vi "Run.vi"(7 "Team Index":i32, 8 "Column":i32, 9 "Row":i32, 10 "View":i32[](array[numeric]) caption="View (Team Index, -1: empty)", 11 "64 In":refnum<class "Picture.lvclass">) -> (0 "Replicated":refnum<class "Square.lvclass">, 1 "Direction":T1, 2 "Action":T2, 3 "64 Out":refnum<class "Picture.lvclass">)   [LabVIEW 2015, in "Picture.lvclass"]
uses:
  Picture.lvclass
  Type Defs/Action Enum.ctl
  Type Defs/Direction Enum.ctl
  Square/Square.lvclass
  Picture.lvclass/Picture.ctl
  SubVIs/Read-Only Globals.vi
  SubVIs/Globals (private).vi
  Type Defs/SB Type Defs.lvlib
  Common/Common.lvlib
panel:
  # "NW\nN\nNE\nE\nSE\nS\nSW\nW"
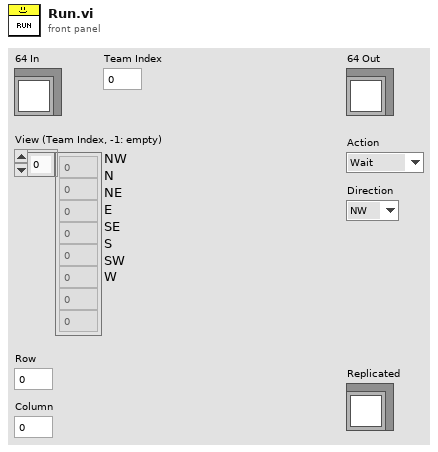
[diagram p1: front panel]
types:
  T1 = typedef "SB Type Defs.lvlib/Direction Enum.ctl" = enum16{"NW", "N", "NE", "E", "SE", "S", "SW", "W"}
  T2 = typedef "SB Type Defs.lvlib/Action Enum.ctl" = enum16{"Wait", "Move", "Attack", "Replicate"}
  T3 = typedef "Common.lvlib/Position.ctl" = cluster{"Column":i32, "Row":i32}
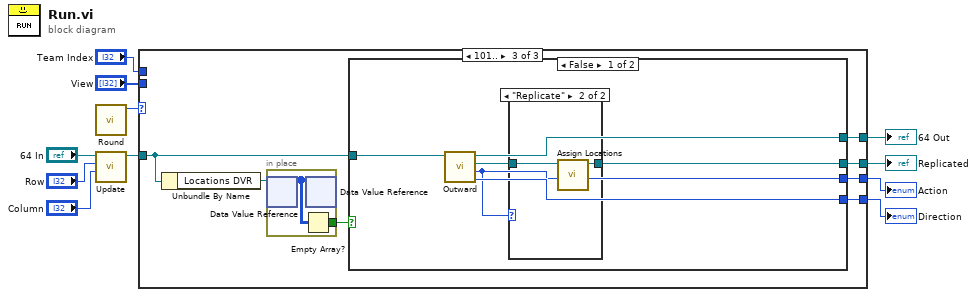
[diagram p0: block diagram]
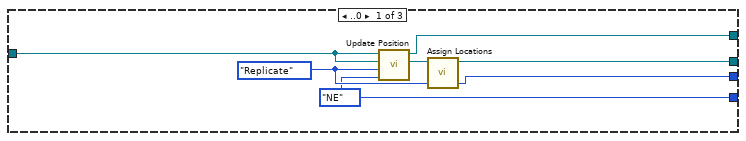
[diagram p2: hidden frame]
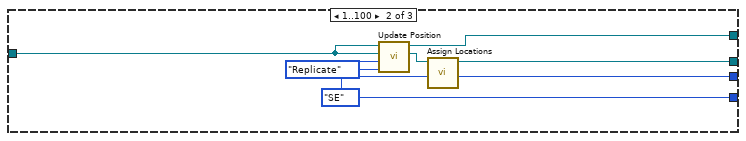
[diagram p3: hidden frame]
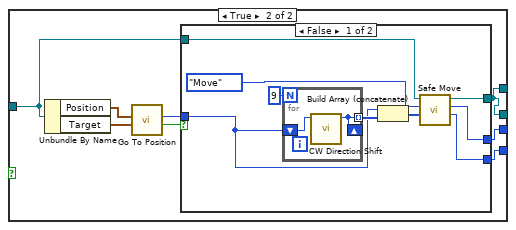
[diagram p5: hidden frame]
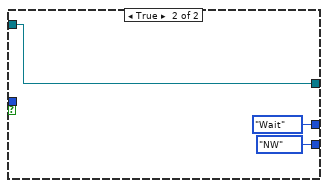
[diagram p6: hidden frame]
diagram:
  n1 = call "Round.vi"() -> ("Round"=w3:i32)  [unwired: 11 in]
  n2 = call "Update.vi"("Column"="Column", "Row"="Row", "64 in"="64 In") -> ("64 out"=w10:refnum<class "Picture.lvclass">)  [unwired: 8 in]
  n3 = case shown="101.." w3 {
    tunnel: w10 -> [w16 w22 w25]
    tunnel: [w15 w21 w30] -> w6
    tunnel: [w12 w18 w28] -> w7
    tunnel: [w14 w20 w27] -> w5
    tunnel: [w13 w19 w29] -> w4
    tunnel: "View" -> [_ _ _]
    tunnel: "Team Index" -> [_ _ _]
    frame ..0 {
      w13 = Direction_Enum."NE" ("Direction")
      w14 = Action_Enum."Replicate" ("Action")
      n4 = call "Update Position.vi"("Direction"=w13, "Action"=w14, "Replicated in"=w16, "64 in"=w16) -> ("Replicated out"=w17:refnum<class "Picture.lvclass">, "64 out"=w15:refnum<class "Picture.lvclass">)  [unwired: 6 in]
      n5 = call "Assign Locations.vi"("Picture In"=w17) -> ("Picture Out"=w12:refnum<class "Picture.lvclass">)  [unwired: 9 in, 1 out]
    }
    frame 1..100 {
      w19 = Direction_Enum."SE" ("Direction")
      w20 = Action_Enum."Replicate" ("Action")
      n6 = call "Update Position.vi"("Direction"=w19, "Action"=w20, "Replicated in"=w22, "64 in"=w22) -> ("Replicated out"=w23:refnum<class "Picture.lvclass">, "64 out"=w21:refnum<class "Picture.lvclass">)  [unwired: 6 in]
      n7 = call "Assign Locations.vi"("Picture In"=w23) -> ("Picture Out"=w18:refnum<class "Picture.lvclass">)  [unwired: 9 in, 1 out]
    }
    frame 101.. {
      n8 = Unbundle By Name(w25) -> ("Locations DVR"=w26:refnum<data-value>)
      n9 = in-place {
        in-place-border: [w62] -> w24
        n10 = in-place-dvr #1(w26) -> (w63:i32[][])  [unwired: 1 out]
        n11 = Empty Array?(array=w63) -> (empty?=w62:bool)
        n12 = in-place-dvr #1(w63) -> ()  [unwired: 2 out]
      }
      n13 = case shown="False" w24 {
        tunnel: [w36 w42] -> w30
        tunnel: [w34 w40] -> w29
        tunnel: [w33 w42] -> w28
        tunnel: [w32 w41] -> w27
        tunnel: w25 -> [w31 w43]
        frame False {
          n14 = call "Outward.vi"("64 in"=w31) -> ("Direction"=w34:i32, "Action"=w32:T2, "Replicated out"=w35:refnum<class "Picture.lvclass">, "64 out"=w36:refnum<class "Picture.lvclass">)  [unwired: 7 in]
          n15 = case shown="\"Replicate\"" w32 {
            tunnel: w35 -> [w37 w39]
            tunnel: [w37 w38] -> w33
            frame Default {
            }
            frame "Replicate" {
              n16 = call "Assign Locations.vi"("Picture In"=w39) -> ("Picture Out"=w38:refnum<class "Picture.lvclass">)  [unwired: 9 in, 1 out]
            }
          }
        }
        frame True {
          n17 = Unbundle By Name(w43) -> ("Position"=w45:T3, "Target"=w46:T3)
          n18 = call "Go To Position.vi"("Target Position"=w46, "My Position"=w45) -> ("Arrived?"=w47:bool, "Direction"=w44:T1)  [unwired: 7 in, 1 out]
          n19 = case shown="False" w47 {
            tunnel: [w56 w61] -> w42
            tunnel: w43 -> [w55 w61]
            tunnel: [w54 Action_Enum."Wait" ("Action out")] -> w41
            tunnel: [w53 Direction_Enum."NW" ("Direction")] -> w40
            tunnel: w44 -> [w49 _]
            frame False {
              n20 = for {
                N: 9 -> [_]
                tunnel: [w57] -> w51 mode=indexing
                shift-right: [w57] -> _
                shift-left: w49 -> [w58]
                n21 = call "CW Direction Shift.vi"("Direction"=w58) -> ("Numeric"=w57:i32)  [unwired: 10 in]
              }
              n22 = Build Array (concatenate)(w49, w51) -> (w50:i32[])
              n23 = call "Safe Move.vi"("Directions in"=w50, "Action in"=Action_Enum."Move", "Picture In"=w55) -> ("Direction"=w53:T1, "Action out"=w54:T2, "Picture Out"=w56:refnum<class "Picture.lvclass">)  [unwired: 5 in, 1 out]
            }
            frame True {
            }
          }
        }
      }
    }
  }
  "64 Out" <- w6
  "Action" <- w5
  "Direction" <- w4
  "Replicated" <- w7
